vi "Endpoint Format.vi"(1 "Endpoint":string="/ShutterOpen", 2 "Channel":i32=1) -> (0 "Endpoint URL":string)   [LabVIEW 2020]
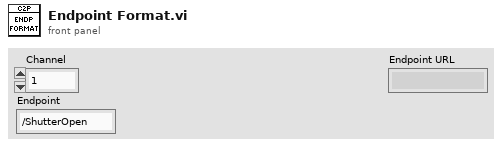
[diagram p1: front panel]
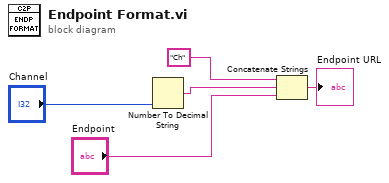
[diagram p0: block diagram]
diagram:
  n1 = Number To Decimal String(number="Channel") -> (decimal integer string=w3:string)  [unwired: 1 in]
  n2 = Concatenate Strings("Ch" ("Endpoint"), w3, "Endpoint") -> (→"Endpoint URL":string)
